vi "Trend_CV.vi"(7 "Original trace (1D)":cluster{"Ramp Pattern":dbl[], "X":dbl[]}[][](array[cluster])) -> (0 "Holding Current (pA)":dbl[](array[numeric]), 3 "CV":dbl[](array[numeric]))   [LabVIEW 2017]
uses:
  <vilib>/Analysis/NI_AALBase.lvlib
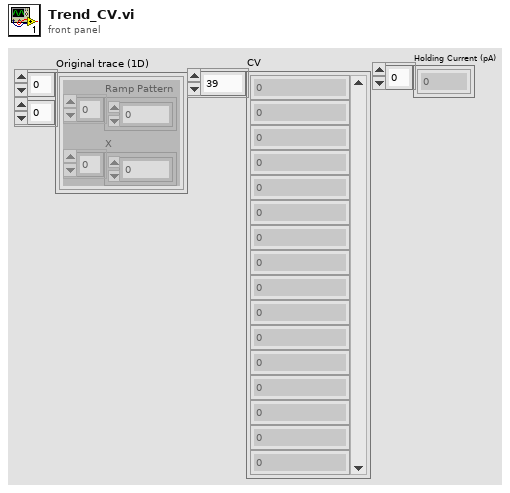
[diagram p1: front panel]
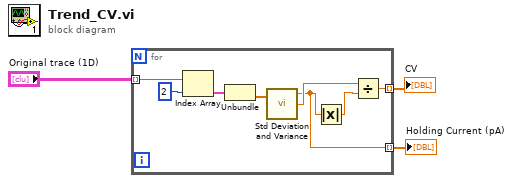
[diagram p0: block diagram]
diagram:
  n1 = for {
    tunnel: "Original trace (1D)" -> [w11] mode=indexing
    tunnel: [w7] -> w2 mode=indexing
    tunnel: [w4] -> w1 mode=indexing
    n2 = Index Array(array=w11, index=2 ("인덱스")) -> (element=w9:cluster{"Ramp Pattern":dbl[], "X":dbl[]})
    n3 = Unbundle(w9) -> ("X"=w6:dbl[])  [unwired: 1 out]
    n4 = call <vilib>:"Std Deviation and Variance.vi"("X"=w6) -> ("mean"=w4:dbl, "standard deviation"=w8:dbl)  [unwired: 1 in, 1 out]
    n5 = Absolute Value(x=w4) -> (abs(x)=w5:dbl)
    n6 = Divide(x=w8, y=w5) -> (x/y=w7:dbl)
  }
  "CV" <- w2
  "Holding Current (pA)" <- w1
